vi "ws Auth Get Expiration Info.vi"(8 "error in (no error)":errorcluster) -> (0 "error out":errorcluster, 2 "Expiration Message":string, 3 "Authorization Expiration Information":T1)   [LabVIEW 2011]
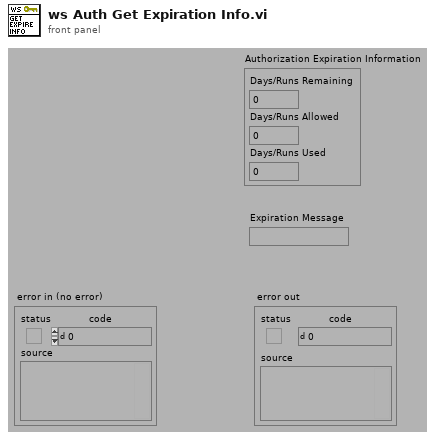
[diagram p1: front panel]
types:
  T1 = cluster{"Days/Runs Remaining":i32, "Days/Runs Allowed":i32, "Days/Runs Used":i32}
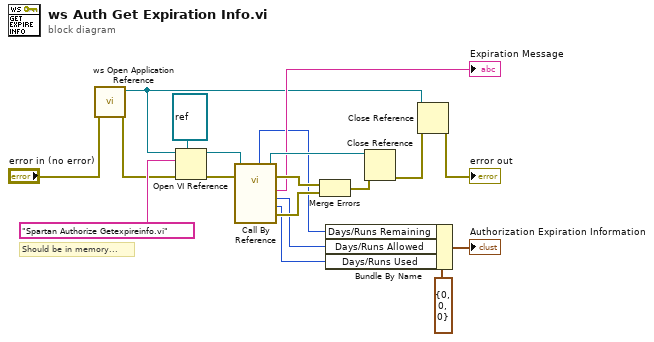
[diagram p0: block diagram]
diagram:
  # "Should be in memory..."
  n1 = call "ws Open Application Reference.vi"("error in (no error)"="error in (no error)") -> ("error out"=w2:errorcluster, "application reference"=w1:refnum<vi>)  [unwired: 9 in]
  n2 = Open VI Reference(type specifier VI Refnum (for type only)=refnum<vi> refnum, application reference (local)=w1, vi path="Spartan Authorize Getexpireinfo.vi", error in (no error)=w2) -> (vi reference=w14:refnum<vi>, error out=w15:errorcluster)  [unwired: 2 in]
  n3 = call-by-ref "?"(reference=w14, error in=w15) -> (reference out=w13:refnum<vi>, error out=w12:errorcluster, 0:"error out"=w11:errorcluster, "Days or runs used"=w5:i32, "Days or Runs allowed"=w6:i32, "Expire Message"=→"Expiration Message":string, "Days/runs remaining"=w8:i32)  [unwired: 7 in]
  n4 = Merge Errors(w12, w11) -> (w17:errorcluster)
  n5 = Bundle By Name(cluster=T1 {"Days/Runs Remaining"=0, "Days/Runs Allowed"=0, "Days/Runs Used"=0} ("Authorization Expiration Information"), "Days/Runs Remaining"=w8, "Days/Runs Allowed"=w6, "Days/Runs Used"=w5) -> (→"Authorization Expiration Information":T1)
  n6 = Close Reference(reference=w13, error in (no error)=w17) -> (error out=w19:errorcluster)
  n7 = Close Reference(reference=w1, error in (no error)=w19) -> (error out=→"error out":errorcluster)
